vi "LibXML_GetAttrNamePtr.vi"(8 "error in":errorcluster, 10 "attribute":u32) -> (0 "error out":errorcluster, 3 "attribute name ptr  out":u32)   [LabVIEW 2019, in "Tools.lvlib" / "LibXML.lvlib"]
doc: "Get attribute name pointer at attrib ptr (U32) input."
uses:
  LibXML.lvlib
  dll/lXMLwrap.dll
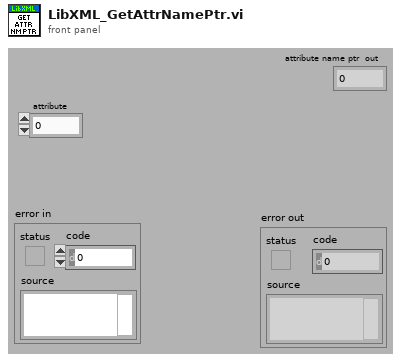
[diagram p1: front panel]
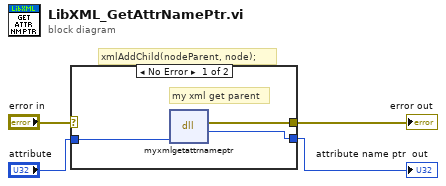
[diagram p0: block diagram]
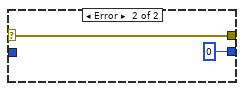
[diagram p2: hidden frame]
diagram:
  # "xmlAddChild(nodeParent, node);"
  n1 = case shown="No Error" "error in" {
    selector: "error in" -> [_ w9]
    tunnel: [w5 w9] -> w3
    tunnel: "attribute" -> [w7 _]
    tunnel: [w6 u32 0 ("return type")] -> w1
    frame No Error {
      # "my xml get parent"
      n2 = dll-call lib="C:/Projects/_Prywatne/MyCIT/Framework/Tools/XML/LibXML/dll/lXMLwrap.dll" fn="myxmlgetattrnameptr"("node"=w7) -> (error out=w5:errorcluster, "return type"=w6:u32)  [unwired: 4 in, 1 out]
    }
    frame Error {
    }
  }
  "error out" <- w3
  "attribute name ptr  out" <- w1
